vi "TDC_getHbtCorrelations.vi"(8 "Error In":errorcluster, 10 "fct in":u64, 11 "forward":bool) -> (0 "Error Out":errorcluster, 3 "fct out":i32)   [LabVIEW 2011]
uses:
  tdcbase.dll
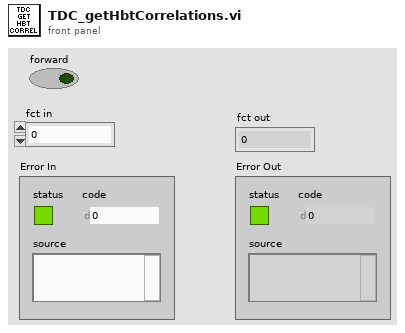
[diagram p1: front panel]
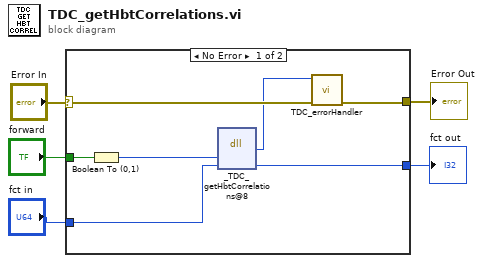
[diagram p0: block diagram]
diagram:
  n1 = case shown="No Error" "Error In" {
    selector: "Error In" -> [w8 w14]
    tunnel: [w7 w14] -> w4
    tunnel: "forward" -> [w10 _]
    tunnel: [w12 w13] -> w2
    tunnel: "fct in" -> [w11 w13]
    frame No Error {
      n2 = Boolean To (0,1)(Boolean=w10) -> (0, 1=w9:i16)
      n3 = dll-call lib="X:/tdcbase.dll" fn="_TDC_getHbtCorrelations@8"("forward"=w9, "fct"=w11) -> ("return type"=w6:i32, "fct"=w12:u64)  [unwired: 4 in, 2 out]
      n4 = call "TDC_errorHandler.vi"("Error In"=w8, "TDC Return Code"=w6) -> ("Error Out"=w7:errorcluster)  [unwired: 9 in]
    }
    frame Error {
    }
  }
  "Error Out" <- w4
  "fct out" <- w2
